vi "Configure IScan Trigger (Measurement Limit).vi"(0 "VISA resource name":refnum<visa-resource-name>, 1 "Limit Test Trigger Source (1: Measurement1)":i32(ring)=1 items=["Measurement1"=1, "Measurement2"=2, "Measurement3"=3, "Measurement4"=4, "Measurement5"=5], 5 "Fail Condition (0: Inside)":i32(ring) items=["Inside", "Outside"], 7 "Lower Limit (-1 s)":dbl=-1.0, 9 "Upper Limit (0 s)":dbl, 11 "error in (no error)":errorcluster) -> (4 "VISA resource name out":refnum<visa-resource-name>, 15 "error out":errorcluster)   [LabVIEW 2020, in "Agilent 90000 Series.lvlib"]
doc: "Configures InfiniiScan trigger under measurement limit trigger mode."
uses:
  Agilent 90000 Series.lvlib
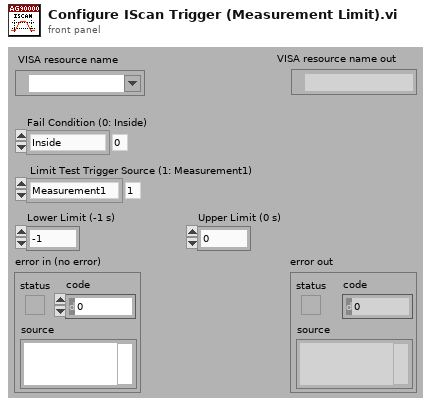
[diagram p1: front panel]
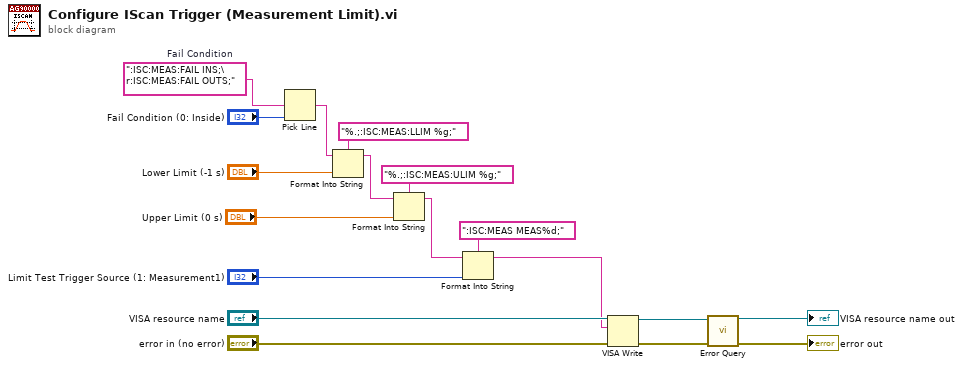
[diagram p0: block diagram]
diagram:
  w18 = ":ISC:MEAS:FAIL INS;\r:ISC:MEAS:FAIL OUTS;"  # Fail Condition
  n1 = Pick Line(multi-line string=w18, line index="Fail Condition (0: Inside)") -> (output string=w1:string)  [unwired: 1 out]
  n2 = Format Into String(format string="%.;:ISC:MEAS:LLIM %g;", initial string=w1, "Lower Limit (-1 s)") -> (resulting string=w4:string)  [unwired: 1 in, 1 out]
  n3 = Format Into String(format string="%.;:ISC:MEAS:ULIM %g;", initial string=w4, "Upper Limit (0 s)") -> (resulting string=w3:string)  [unwired: 1 in, 1 out]
  n4 = Format Into String(format string=":ISC:MEAS MEAS%d;", initial string=w3, "Limit Test Trigger Source (1: Measurement1)") -> (resulting string=w2:string)  [unwired: 1 in, 1 out]
  n5 = VISA Write(VISA resource name="VISA resource name", write buffer=w2, error in (no error)="error in (no error)") -> (VISA resource name out=w9:refnum<visa-resource-name>, error out=w8:errorcluster)  [unwired: 1 out]
  n6 = call "Error Query.vi"("error in (no error)"=w8, "VISA resource name"=w9) -> ("error out"=→"error out":errorcluster, "VISA resource name out"=→"VISA resource name out":refnum<visa-resource-name>)  [unwired: 8 out]
